vi "MetrolabRead.vi"(3 "Input string":string="ENQ,3\r", 4 "error in (no error)":errorcluster caption="エラー入力（エラーなし）", 5 "VISA resource name":refnum<visa-resource-name>="COM5") -> (0 "B value [mT]":dbl, 1 "String":string="\r\n", 2 "error out":errorcluster caption="エラー出力" {"code" format="%.0x"})   [LabVIEW 2017]
uses:
  <vilib>/Instr/_visa.llb/VISA Configure Serial Port (Serial Instr).vi
panel:
  # "Metrolab THM7025"
  # "Pressure\nB value [mT]"
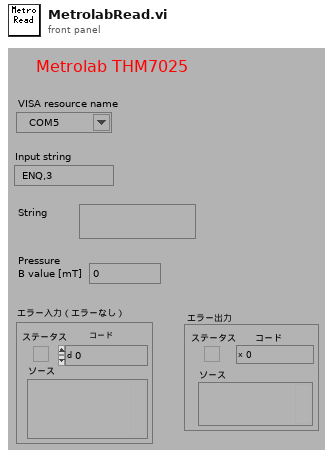
[diagram p1: front panel]
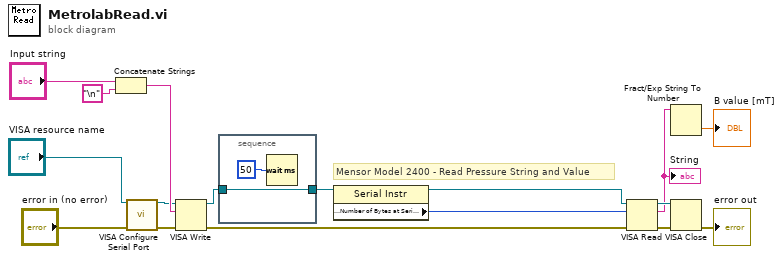
[diagram p0: block diagram]
diagram:
  # "Mensor Model 2400 - Read Pressure String and Value"
  n1 = Concatenate Strings("Input string", "\n") -> (w13:string)
  n2 = call-poly "VISA Configure Serial Port"("VISA resource name"="VISA resource name", "error in (no error)"="error in (no error)") -> ("VISA resource name out"=w8:refnum<visa-resource-name>, "error out"=w10:errorcluster)  [unwired: 12 in]
  n3 = VISA Write(VISA resource name=w8, write buffer=w13, error in (no error)=w10) -> (VISA resource name out=w14:refnum<visa-resource-name>, error out=w11:errorcluster)  [unwired: 1 out]
  n4 = stacked-sequence {
    tunnel: w14 -> [w18]
    tunnel: [w18] -> w15
    frame #0 {
      n5 = Wait (ms)(milliseconds to wait=50) -> ()  [unwired: 1 out]
    }
  }
  n6 = property class="Serial Instr"(reference=w15) -> (reference out=w16:refnum<visa-resource-name>, "Serial Settings:Number of Bytes at Serial Port"=w17:u32)  [unwired: 1 in, 1 out]
  n7 = VISA Read(VISA resource name=w16, byte count=w17, error in (no error)=w11) -> (VISA resource name out=w9:refnum<visa-resource-name>, read buffer=w5:string, error out=w12:errorcluster)  [unwired: 1 out]
  "String" <- w5
  n8 = Fract/Exp String To Number(string=w5) -> (number=→"B value [mT]":dbl)  [unwired: 3 in, 1 out]
  n9 = VISA Close(VISA resource name=w9, error in (no error)=w12) -> (error out=→"error out":errorcluster)
